vi "PhotonTrackedTarget_GetYaw.vi"(11 "TrackedTarget":T1={"Yaw"=0.0, "Pitch"=0.0, "Area"=0.0, "Skew"=0.0, "MinAreaRectCorners"=[], "BestCameraToTarget"={"TRANSLATION3D"={"X"=0.0, "Y"=0.0, "Z"=0.0}, "ROTATION3D"={"Q_quaternion"={"R"=1.0, "V"=[0.0, 0.0, 0.0]}}, "XF"=FALSE}, "FiducialId"=0, "AltCameraToTarget"={"TRANSLATION3D"={"X"=0.0, "Y"=0.0, "Z"=0.0}, "ROTATION3D"={"Q_quaternion"={"R"=1.0, "V"=[0.0, 0.0, 0.0]}}, "XF"=FALSE}, "PoseAmbiguity"=0.0, "DetectedCorners"=[], "ObjDetectId"=0, "ObjDetectConf"=0.0} {"AltCameraToTarget"."TRANSLATION3D"."Z" format="%14.3f"; "AltCameraToTarget"."TRANSLATION3D"."Y" format="%14.3f"; "AltCameraToTarget"."TRANSLATION3D"."X" format="%14.3f"; "BestCameraToTarget"."TRANSLATION3D"."Z" format="%14.3f"; "BestCameraToTarget"."TRANSLATION3D"."Y" format="%14.3f"; "BestCameraToTarget"."TRANSLATION3D"."X" format="%14.3f"}) -> (3 "Yaw":dbl)   [LabVIEW 2019, in "PhotonVisionLib.lvlib"]
doc: "Get Yaw from Tracked Target\n\nInputs:\n - TrackedTarget -- Parsed TrackedTarget cluster.\n\nOutputs:\n - Yaw -- Yaw value"
uses:
  PhotonVisionLib.lvlib
  TypeDef/PhotonTrackedTargetType.ctl
  TypeDef/TargetCornerType.ctl
  <vilib>/Rock Robotics/WPI/ThirdParty/JAS_Junk/TrajLib/TypeDef/TRANSFORM3D.ctl
  <vilib>/Rock Robotics/WPI/ThirdParty/JAS_Junk/TrajLib/TypeDef/TRANSLATION3D.ctl
  <vilib>/Rock Robotics/WPI/ThirdParty/JAS_Junk/TrajLib/TypeDef/ROTATION3D.ctl
  <vilib>/Rock Robotics/WPI/ThirdParty/JAS_Junk/TrajLib/TypeDef/QUATERNION.ctl
  <vilib>/Rock Robotics/WPI/ThirdParty/JAS_Junk/TrajLib/Trajectory_Library.lvlib
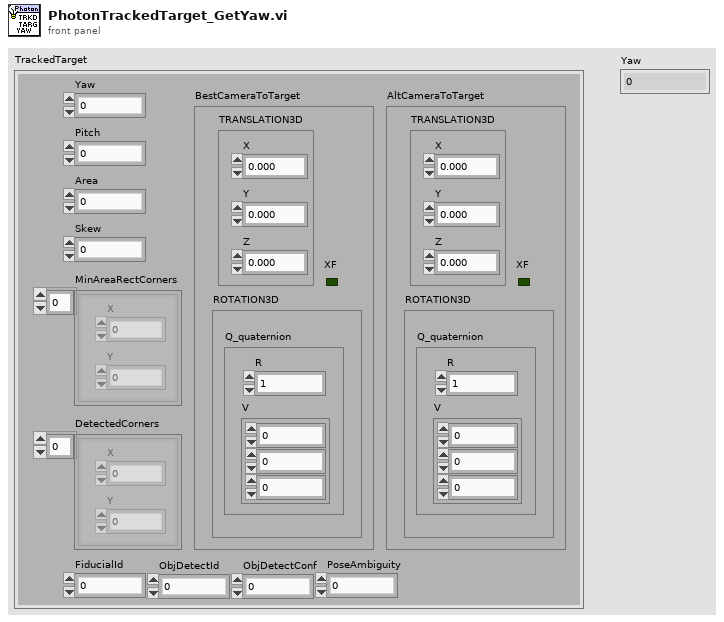
[diagram p1: front panel]
types:
  T1 = typedef "PhotonVisionLib.lvlib/PhotonTrackedTargetType.ctl" = cluster{"Yaw":dbl, "Pitch":dbl, "Area":dbl, "Skew":dbl, "MinAreaRectCorners":T2[], "BestCameraToTarget":T3, "FiducialId":i32, "AltCameraToTarget":T3, "PoseAmbiguity":dbl, "DetectedCorners":T2[], "ObjDetectId":i32, "ObjDetectConf":sgl}
  T2 = typedef "PhotonVisionLib.lvlib/TargetCornerType.ctl" = cluster{"X":dbl, "Y":dbl}
  T3 = typedef "Trajectory_Library.lvlib/TRANSFORM3D.ctl" = cluster{"TRANSLATION3D":T4, "ROTATION3D":T5, "XF":bool}
  T4 = typedef "Trajectory_Library.lvlib/TRANSLATION3D.ctl" = cluster{"X":dbl, "Y":dbl, "Z":dbl}
  T5 = typedef "Trajectory_Library.lvlib/ROTATION3D.ctl" = cluster{"Q_quaternion":T6}
  T6 = typedef "Trajectory_Library.lvlib/QUATERNION.ctl" = cluster{"R":dbl, "V":dbl[]}
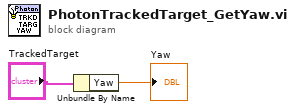
[diagram p0: block diagram]
diagram:
  n1 = Unbundle By Name("TrackedTarget") -> ("Yaw"=→"Yaw":dbl)
